vi "Delete DVR.vi"(8 "error in (no error)":errorcluster, 11 "data value reference":refnum<data-value>) -> (0 "error out":errorcluster, 3 "Motor Obj":refnum<class "Motor.lvclass">)   [LabVIEW 2016, in "Hardware.lvlib" / "Motor.lvlib" / "Motor.lvclass"]
uses:
  <userlib>/Common Components/Hardware/Motor/Motor/Motor.lvclass
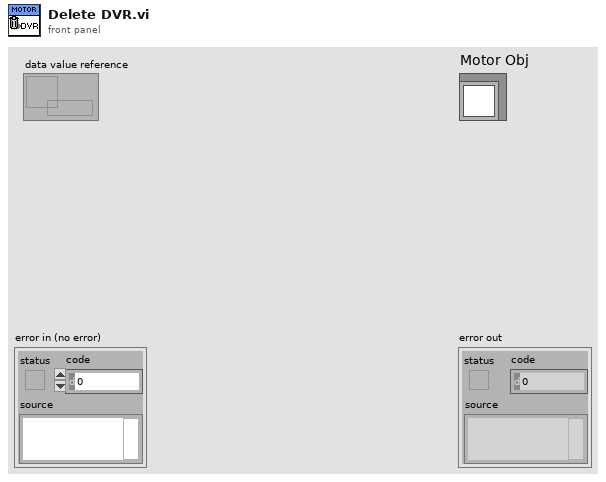
[diagram p1: front panel]
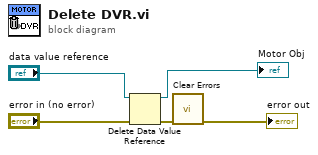
[diagram p0: block diagram]
diagram:
  n1 = Delete Data Value Reference(data value reference="data value reference", error in="error in (no error)") -> (data value=→"Motor Obj":refnum<class "Motor.lvclass">, error out=w3:errorcluster)
  n2 = call <vilib>:"Clear Errors.vi"("error in (no error)"=w3) -> ("error out"=→"error out":errorcluster)  [unwired: 5 in, 1 out]
